vi "Initialise CAN Interface.vi"(8 "error in (no error)":errorcluster, 11 "CAN Frame Sessions":T1={"Session_Control"="Sess_Control", "Session_Params"="Sess_Params", "Session_Actuals"="Sess_Actuals", "Session_Acknowledge"="Sess_Ack", "Session_H2_Sensor"="H2_Sensor_Session", "Session_DILICO_MeasurementRequest"="Session_DILICO_MeasurementRequest", "Session_DILICO_Voltages"="Session_DILICO_Voltages"}) -> (0 "error out":errorcluster={"status"=TRUE, "code"=-1074384864, "source"="XNET Write (Signal Single-point).vi:3310001<APPEND>\n\n<b>Complete call chain:</b>\r\n     XNET Write (Signal Single-point).vi:3310001\r\n     phlair-busch-can-bus.lvlib:Initialise Interface.vi"}, 3 "output cluster":T1={"Session_Control"="Session_Control", "Session_Params"="Session_Params", "Session_Actuals"="Session_Actuals", "Session_Acknowledge"="Session_Acknowledge", "Session_H2_Sensor"="H2_Sensor_Session", "Session_DILICO_MeasurementRequest"="H2_Sensor_Session", "Session_DILICO_Voltages"="H2_Sensor_Session"})   [LabVIEW 2025, in "phlair-busch-can-bus.lvlib"]
uses:
  phlair-busch-can-bus.lvlib
  CAN Frame Sessions.ctl
  <userlib>/_OpenG.lib/error/error.llb/openg_error.lvlib
  <resource>/objmgr/xnet.rc
panel:
  out "Session_DILICO_Voltages":refnum<k21>
  out "Session_DILICO_MeasurementRequest":refnum<k21>
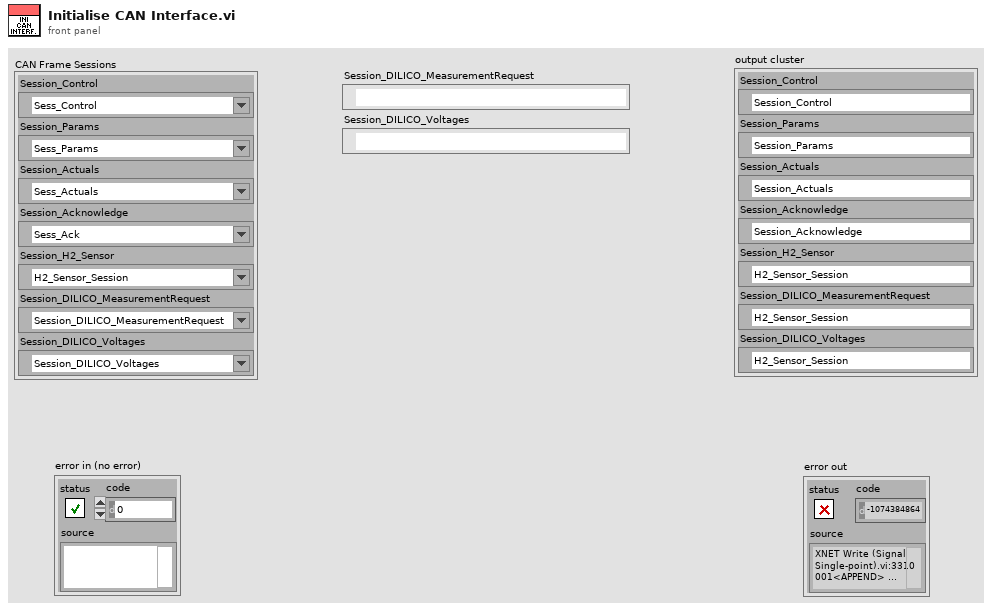
[diagram p1: front panel]
types:
  T1 = typedef "phlair-busch-can-bus.lvlib/CAN Frame Sessions.ctl" = cluster{"Session_Control":refnum<k21>, "Session_Params":refnum<k21>, "Session_Actuals":refnum<k21>, "Session_Acknowledge":refnum<k21>, "Session_H2_Sensor":refnum<k21>, "Session_DILICO_MeasurementRequest":refnum<k21>, "Session_DILICO_Voltages":refnum<k21>}
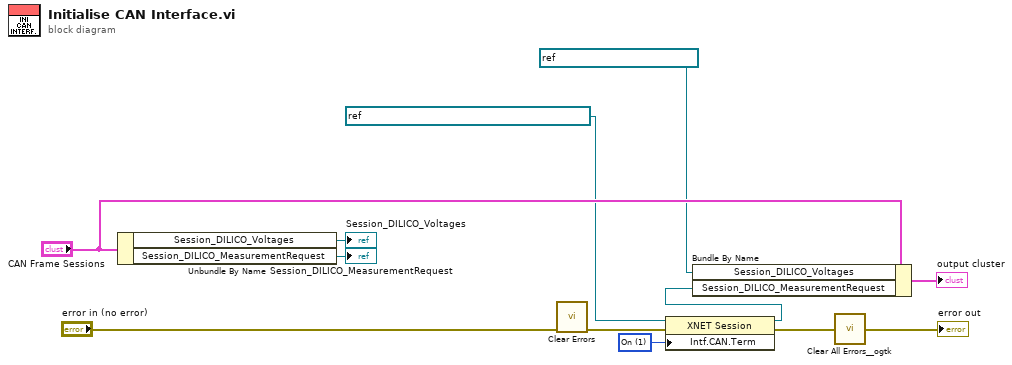
[diagram p0: block diagram]
diagram:
  w12 = u32 1 items=["Off", "On"] ("Interface:CAN:Termination")
  n1 = Unbundle By Name("CAN Frame Sessions") -> ("Session_DILICO_Voltages"=→"Session_DILICO_Voltages":refnum<k21>, "Session_DILICO_MeasurementRequest"=→"Session_DILICO_MeasurementRequest":refnum<k21>)
  n2 = call <vilib>:"Clear Errors.vi"("error in (no error)"="error in (no error)") -> ("error out"=w7:errorcluster)  [unwired: 5 in, 1 out]
  n3 = property class="XNET Session"(reference=refnum<k21> "Session_DILOCO_MeasurementRequest" ("XNET Session"), error in=w7, "Intf.CAN.Term"=w12) -> (reference out=w6:refnum<k21>, error out=w10:errorcluster)
  n4 = Bundle By Name(cluster="CAN Frame Sessions", "Session_DILICO_Voltages"=refnum<k21> "Session_DILICO_Voltages", "Session_DILICO_MeasurementRequest"=w6) -> (→"output cluster":T1)
  n5 = call <userlib>:"Clear All Errors__ogtk.vi"("Error In"=w10) -> ("Error Out"=→"error out":errorcluster)  [unwired: 3 in]
